vi "get action display names.vi"(8 "error in (no error)":errorcluster, 10 "supported actions list":T1[](array[typedef]), 11 "action configs":refnum<class "action configuration.lvclass">[](array[class])) -> (0 "error out":errorcluster, 3 "display names":string[](array[string]))   [LabVIEW 2014, in "Simple Sequencer TBM editor node.lvclass"]
doc: "This returns an array of display names for a given array of actions."
uses:
  Simple Sequencer TBM editor node.lvclass
  sequencer parent classes/action configuration parent/action configuration.lvclass
  action config and UI pairing.ctl
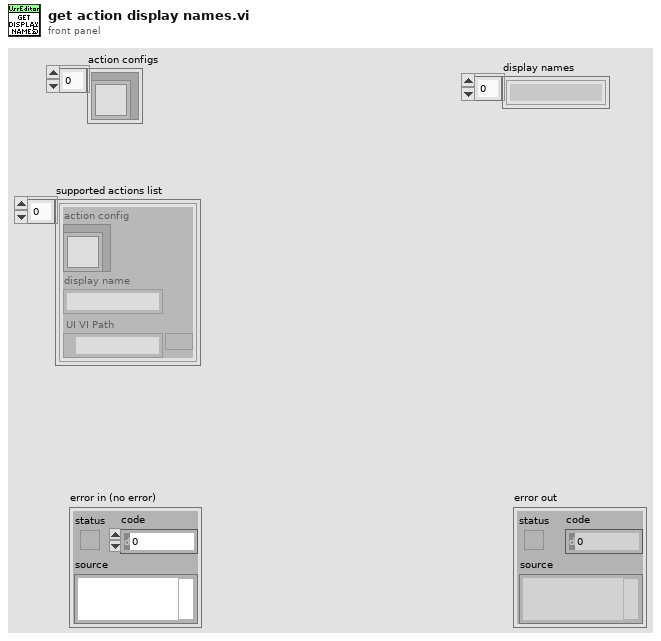
[diagram p1: front panel]
types:
  T1 = typedef "Simple Sequencer TBM editor node.lvclass/action config and UI pairing.ctl" = cluster{"action config":refnum<class "action configuration.lvclass">, "display name":string, "UI VI Path":path}
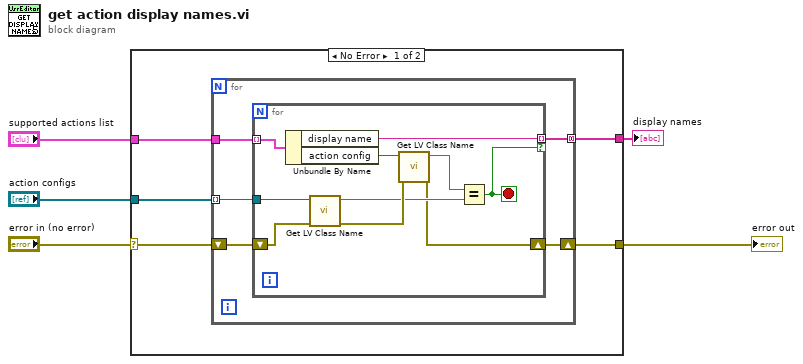
[diagram p0: block diagram]
diagram:
  n1 = case shown="No Error" "error in (no error)" {
    selector: "error in (no error)" -> [w8 w26]
    tunnel: [w6 w26] -> w4
    tunnel: "supported actions list" -> [w9 _]
    tunnel: "action configs" -> [w10 _]
    tunnel: [w7 _] -> w2
    frame No Error {
      n2 = for {
        tunnel: w10 -> [w14] mode=indexing
        tunnel: w9 -> [w15]
        shift-right: [w12] -> w6
        shift-left: w8 -> [w13]
        tunnel: [w11] -> w7 mode=concatenating
        n3 = for {
          tunnel: w15 -> [w24] mode=indexing
          tunnel: w14 -> [w25]
          shift-right: [w18] -> w12
          shift-left: w13 -> [w23]
          tunnel: [w17] -> w11 mode=indexing if=w16
          stop <- w16 stop-if-true
          n4 = Unbundle By Name(w24) -> ("display name"=w17:string, "action config"=w21:refnum<class "action configuration.lvclass">)
          n5 = call <vilib>:"Get LV Class Name.vi"("error in (no error)"=w23, "object"=w25) -> ("error out"=w22:errorcluster, "class name"=w20:string)  [unwired: 8 in]
          n6 = call <vilib>:"Get LV Class Name.vi"("error in (no error)"=w22, "object"=w21) -> ("error out"=w18:errorcluster, "class name"=w19:string)  [unwired: 8 in]
          n7 = Equal?(x=w19, y=w20) -> (x = y?=w16:bool)
        }
      }
    }
    frame Error {
    }
  }
  "error out" <- w4
  "display names" <- w2
